vi "bwStimulus.vi"(8 "error in (no error)":errorcluster, 11 "Stimulus in":refnum<class "Stimulus.lvclass">) -> (0 "error out":errorcluster, 3 "Stimulus out":refnum<class "Stimulus.lvclass">)   [LabVIEW 2013]
uses:
  Stimulus.lvclass
panel:
  in  "ITI":u32=2000
  in  "current time 2":timestamp
  out "current time":timestamp
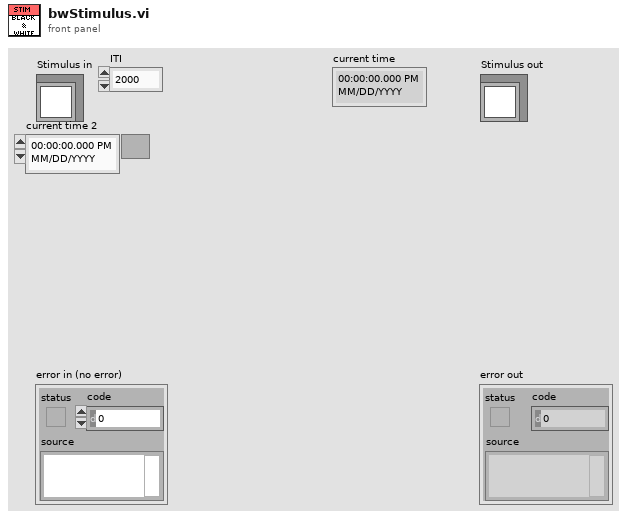
[diagram p1: front panel]
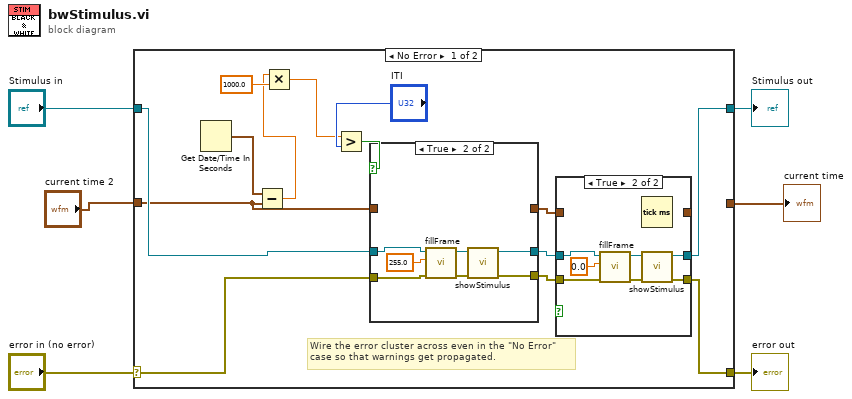
[diagram p0: block diagram]
diagram:
  n1 = case shown="No Error" "error in (no error)" {
    selector: "error in (no error)" -> [w13 w43]
    tunnel: [w12 w43] -> w5
    tunnel: [w14 w42] -> w3
    tunnel: "Stimulus in" -> [w15 w42]
    tunnel: "current time 2" -> [w10 w41]
    tunnel: [_ w41] -> w1
    frame No Error {
      # "Wire the error cluster across even in the \"No Error\"\ncase so that warnings get propagated."
      n2 = Get Date/Time In Seconds() -> (seconds since 1Jan1904=w11:timestamp)
      n3 = Subtract(x=w11, y=w10) -> (x-y=w8:dbl)
      n4 = Multiply(x=w8, y=1000.0) -> (x*y=w7:dbl)
      n5 = Greater?(x=w7, y="ITI") -> (0:w19:bool)
      n6 = case shown="True" w19 {
        tunnel: w15 -> [w33 w40]
        tunnel: [w33 w39] -> w18
        tunnel: [w31 w38] -> w17
        tunnel: w10 -> [w32 _]
        tunnel: [w32 _] -> w16
        tunnel: w13 -> [w31 w34]
        frame False {
        }
        frame True {
          n7 = call-dynamic "fillFrame.vi"("error in (no error)"=w34, "Pixel Value (U8, U16, I16, Float)"=sgl 255.0, "Stimulus in"=w40) -> ("error out"=w35:errorcluster, "Stimulus out"=w37:refnum<class "Stimulus.lvclass">)  [unwired: 7 in]
          n8 = call-dynamic "showStimulus.vi"("error in (no error)"=w35, "Stimulus in"=w37) -> ("error out"=w38:errorcluster, "Stimulus out"=w39:refnum<class "Stimulus.lvclass">)  [unwired: 8 in]
        }
      }
      n9 = case shown="True" {
        selector: _ -> [_ _]
        tunnel: w18 -> [w23 w27]
        tunnel: [w23 w26] -> w14
        tunnel: w17 -> [w22 w25]
        tunnel: [w22 w24] -> w12
        tunnel: [w21 _] -> _
        tunnel: w16 -> [w21 _]
        frame False {
        }
        frame True {
          n10 = call-dynamic "fillFrame.vi"("error in (no error)"=w25, "Pixel Value (U8, U16, I16, Float)"=sgl 0.0, "Stimulus in"=w27) -> ("error out"=w28:errorcluster, "Stimulus out"=w30:refnum<class "Stimulus.lvclass">)  [unwired: 7 in]
          n11 = Tick Count (ms)() -> ()  [unwired: 1 out]
          n12 = call-dynamic "showStimulus.vi"("error in (no error)"=w28, "Stimulus in"=w30) -> ("error out"=w24:errorcluster, "Stimulus out"=w26:refnum<class "Stimulus.lvclass">)  [unwired: 8 in]
        }
      }
    }
    frame Error {
    }
  }
  "error out" <- w5
  "Stimulus out" <- w3
  "current time" <- w1
